vi "Day12-validate_path.vi"(11 "Path":string[](array[string])) -> (1 "invalid?":bool, 2 "finshed?":bool, 3 "Path out":string[](array[string]))   [LabVIEW 2021]
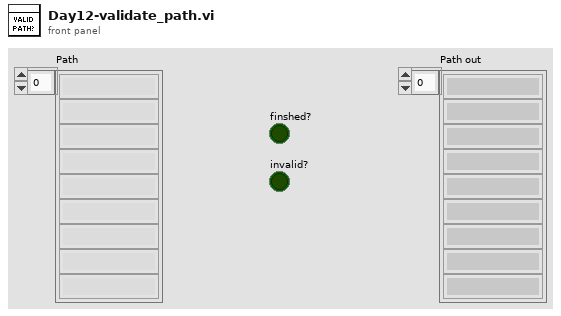
[diagram p1: front panel]
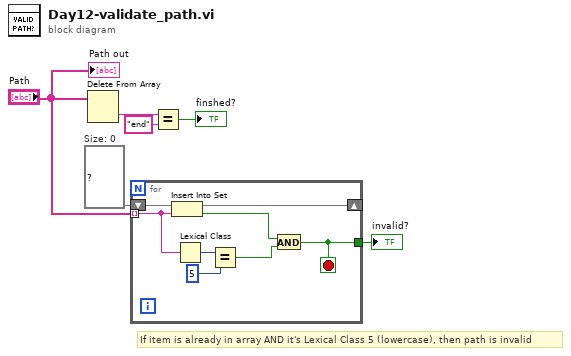
[diagram p0: block diagram]
diagram:
  w3 = set{string} {}  # Size: 0
  # "If item is already in array AND it's Lexical Class 5 (lowercase), then path is invalid"
  n1 = Delete From Array(array="Path") -> (deleted portion=w6:string)  [unwired: 2 in, 1 out]
  n2 = for {
    tunnel: "Path" -> [w12] mode=indexing
    shift-right: [w14] -> _
    shift-left: w3 -> [w13]
    tunnel: [w7] -> w2
    stop <- w7 stop-if-true
    n3 = Insert Into Set(10:w12, 11:w13) -> (2:w9:bool, 3:w14:set{string})
    n4 = Lexical Class(1:w12) -> (0:w11:i16)
    n5 = Equal?(x=w11, y=i16 5) -> (x = y?=w8:bool)
    n6 = And(x=w9, y=w8) -> (x .and. y?=w7:bool)
  }
  "invalid?" <- w2
  n7 = Equal?(x=w6, y="end") -> (x = y?=→"finshed?":bool)
  "Path out" <- "Path"
